vi "Get Virt Instr.vi"(8 "error in (no error)":errorcluster, 11 "Host Measure and Stimulus Subsystems in":refnum<class "Measure and Stimulus Subsystems.lvclass">) -> (0 "error out":errorcluster, 2 "Virt Instr":T1(c390), 3 "Host Measure and Stimulus Subsystems out":refnum<class "Measure and Stimulus Subsystems.lvclass">)   [LabVIEW 2023, in "HAL GOOP4.lvlib" / "Measure and Stimulus Subsystems.lvclass"]
uses:
  Measure and Stimulus Subsystems.lvclass
  Virt Instr Host/Virt Instr Host.lvclass
  Measure and Stimulus Subsystems.lvclass/Measure and Stimulus Subsystems.ctl
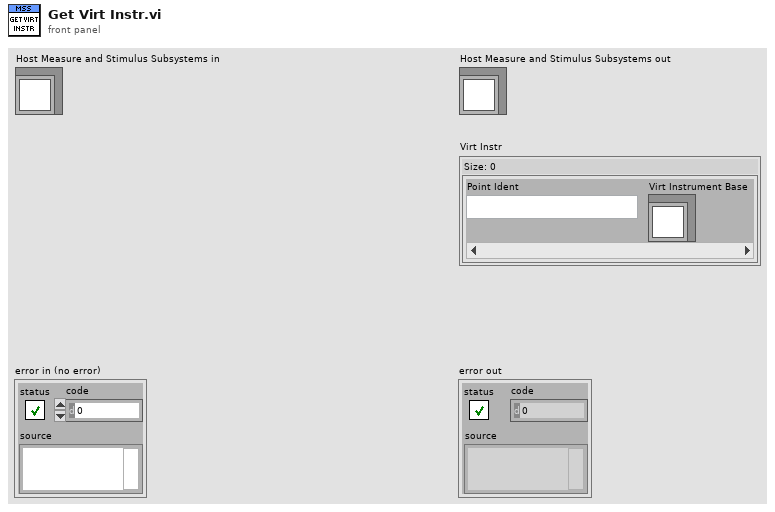
[diagram p1: front panel]
types:
  T1 = map{string, refnum<class "Virt Instr Host.lvclass">}
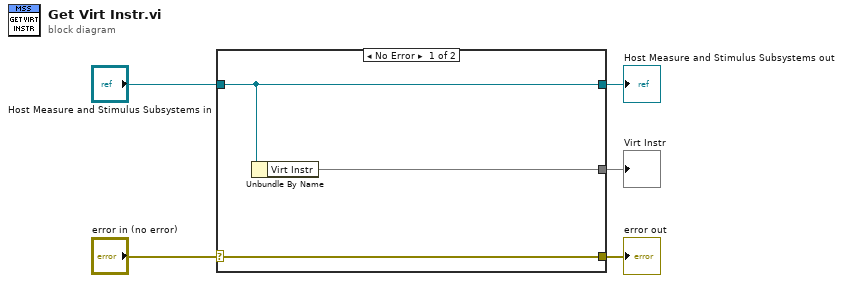
[diagram p0: block diagram]
diagram:
  n1 = case shown="No Error" "error in (no error)" {
    selector: "error in (no error)" -> [w8 w9]
    tunnel: [w8 w9] -> w4
    tunnel: [w7 w10] -> w2
    tunnel: "Host Measure and Stimulus Subsystems in" -> [w7 w10]
    tunnel: [w6 _] -> w1
    frame No Error {
      n2 = Unbundle By Name(w7) -> ("Virt Instr"=w6:T1)
    }
    frame Error {
    }
  }
  "error out" <- w4
  "Host Measure and Stimulus Subsystems out" <- w2
  "Virt Instr" <- w1
